vi "QCA Change Channels.vi"(0 "Channel":i32) -> ()   [LabVIEW 2010]
uses:
  QCA Global.vi
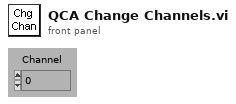
[diagram p1: front panel]
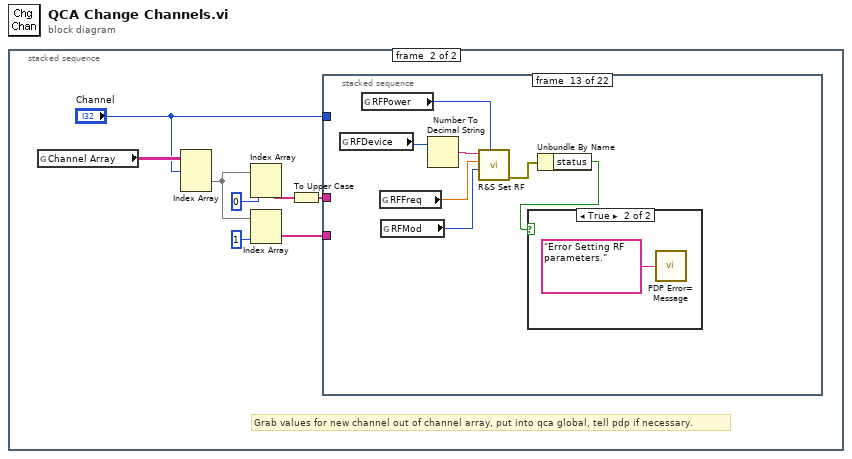
[diagram p0: block diagram]
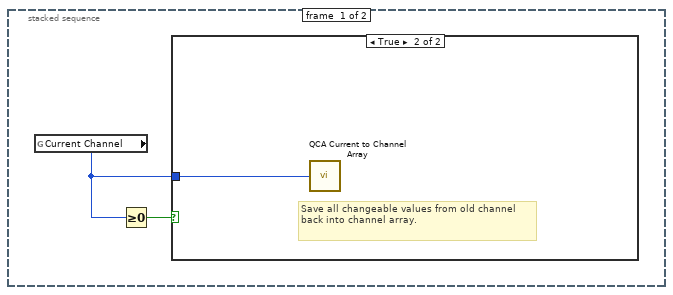
[diagram p2: hidden frame]
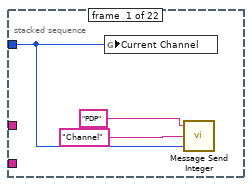
[diagram p4: hidden frame]
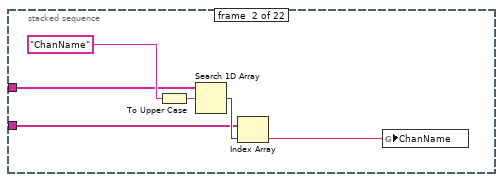
[diagram p5: hidden frame]
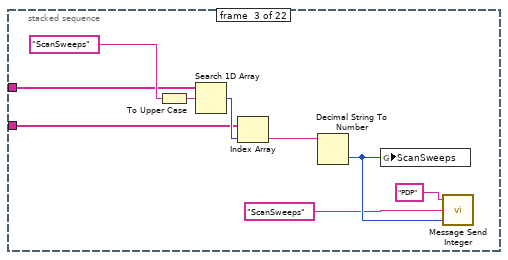
[diagram p6: hidden frame]
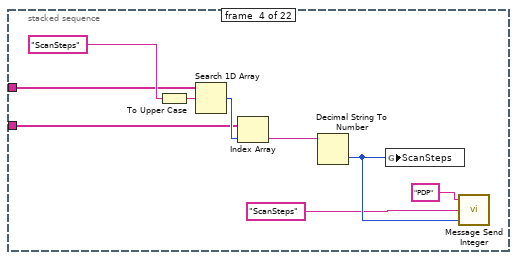
[diagram p7: hidden frame]
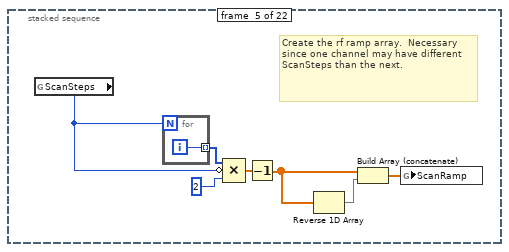
[diagram p8: hidden frame]
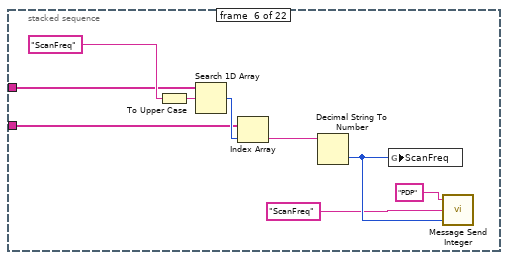
[diagram p9: hidden frame]
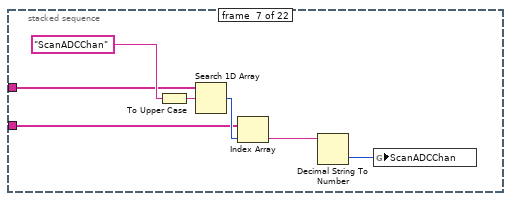
[diagram p10: hidden frame]
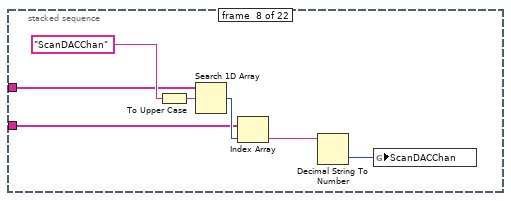
[diagram p11: hidden frame]
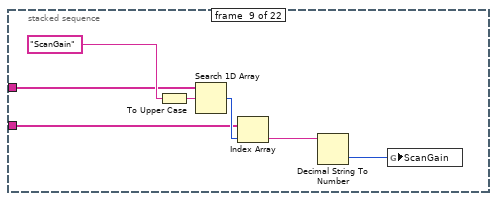
[diagram p12: hidden frame]
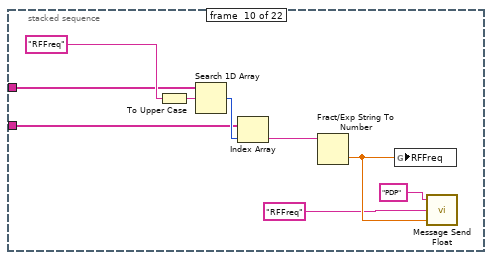
[diagram p13: hidden frame]
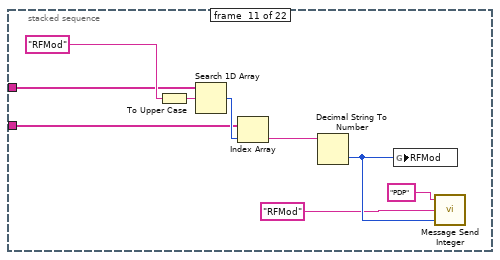
[diagram p14: hidden frame]
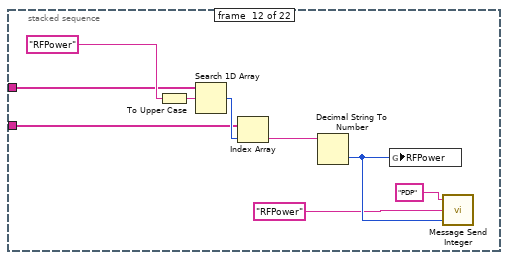
[diagram p15: hidden frame]
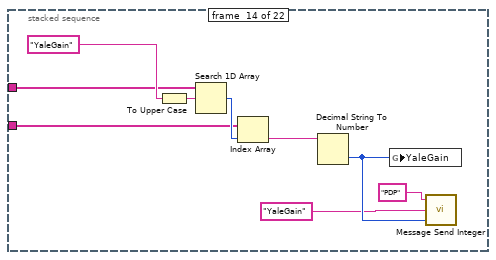
[diagram p17: hidden frame]
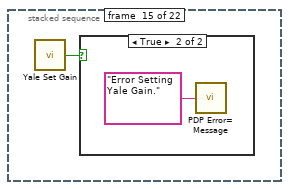
[diagram p18: hidden frame]
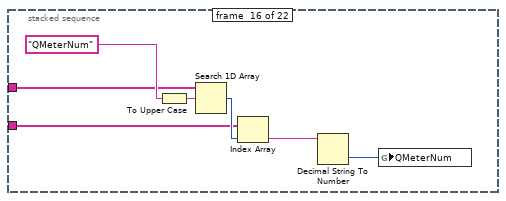
[diagram p20: hidden frame]
diagram:
  n1 = stacked-sequence {
    frame #0 {
      n2 = global read "QCA Global.vi" "Current Channel"() -> (w1:i32)
      n3 = Greater Or Equal To 0?(x=w1) -> (x >= 0?=w2:bool)
      n4 = case shown="True" w2 {
        tunnel: w1 -> [_ w3]
        frame False {
        }
        frame True {
          # "Save all changeable values from old channel back into channel array."
          n5 = call "QCA Current to Channel Array.vi"("Channel Number"=w3) -> ()
        }
      }
    }
    frame #1 {
      # "Grab values for new channel out of channel array, put into qca global, tell pdp if necessary."
      n6 = global read "QCA Global.vi" "Channel Array"() -> (w10:string[][][])
      n7 = Index Array(array=w10, index (dim 0)="Channel") -> (element=w6:string[][])  [unwired: 2 in]
      n8 = Index Array(array=w6, index (col)=0 ("Index")) -> (element=w9:string[])  [unwired: 1 in]
      n9 = Index Array(array=w6, index (col)=1 ("Index")) -> (element=w7:string[])  [unwired: 1 in]
      n10 = To Upper Case(1:w9) -> (0:w4:string[])
      n11 = stacked-sequence {
        tunnel: w4 -> [_ w17 w26 w35 _ w52 w59 w66 w73 w82 w91 w100 _ w117 _ w126 w134 _ w145 w155 w166 w173]
        tunnel: w7 -> [_ w16 w25 w34 _ w51 w58 w65 w72 w81 w90 w99 _ w116 _ w125 w133 _ w144 w154 w165 w172]
        tunnel: "Channel" -> [w14 _ _ _ _ _ _ _ _ _ _ _ _ _ _ _ _ _ _ _ _ _]
        frame #0 {
          n12 = global write "QCA Global.vi" "Current Channel"(w14) -> ()
          n13 = call "Message Send Integer.vi"("Value"=w14, "Parameter"="Channel", "Destination"="PDP") -> ()
        }
        frame #1 {
          n14 = To Upper Case(1:"ChanName" ("element")) -> (0:w18:string)
          n15 = Search 1D Array(1D array=w17, element=w18) -> (index of element=w19:i32)  [unwired: 1 in]
          n16 = Index Array(array=w16, index=w19) -> (element=w15:string)
          n17 = global write "QCA Global.vi" "ChanName"(w15) -> ()
        }
        frame #2 {
          n18 = To Upper Case(1:"ScanSweeps" ("element")) -> (0:w27:string)
          n19 = Search 1D Array(1D array=w26, element=w27) -> (index of element=w28:i32)  [unwired: 1 in]
          n20 = Index Array(array=w25, index=w28) -> (element=w24:string)
          n21 = Decimal String To Number(string=w24) -> (number=w23:i32)  [unwired: 2 in, 1 out]
          n22 = global write "QCA Global.vi" "ScanSweeps"(w23) -> ()
          n23 = call "Message Send Integer.vi"("Value"=w23, "Parameter"="ScanSweeps", "Destination"="PDP") -> ()
        }
        frame #3 {
          n24 = To Upper Case(1:"ScanSteps" ("element")) -> (0:w36:string)
          n25 = Search 1D Array(1D array=w35, element=w36) -> (index of element=w37:i32)  [unwired: 1 in]
          n26 = Index Array(array=w34, index=w37) -> (element=w33:string)
          n27 = Decimal String To Number(string=w33) -> (number=w32:i32)  [unwired: 2 in, 1 out]
          n28 = global write "QCA Global.vi" "ScanSteps"(w32) -> ()
          n29 = call "Message Send Integer.vi"("Value"=w32, "Parameter"="ScanSteps", "Destination"="PDP") -> ()
        }
        frame #4 {
          # "Create the rf ramp array.  Necessary since one channel may have different ScanSteps than the next."
          n30 = global read "QCA Global.vi" "ScanSteps"() -> (w42:i32)
          n31 = for {
            N: w42 -> [_]
            tunnel: [w46] -> w45 mode=indexing
            i -> [w46]
          }
          n32 = Compound Arithmetic op=MULTIPLY(w45, invert w42, 2 ("Input")) -> (w43:dbl[])
          n33 = Decrement(x=w43) -> (x-1=w40:dbl[])
          n34 = Reverse 1D Array(array=w40) -> (reversed array=w41:dbl[])
          n35 = Build Array (concatenate)(w40, w41) -> (w39:dbl[])
          n36 = global write "QCA Global.vi" "ScanRamp"(w39) -> ()
        }
        frame #5 {
          n37 = To Upper Case(1:"ScanFreq" ("element")) -> (0:w53:string)
          n38 = Search 1D Array(1D array=w52, element=w53) -> (index of element=w54:i32)  [unwired: 1 in]
          n39 = Index Array(array=w51, index=w54) -> (element=w50:string)
          n40 = Decimal String To Number(string=w50) -> (number=w49:i32)  [unwired: 2 in, 1 out]
          n41 = global write "QCA Global.vi" "ScanFreq"(w49) -> ()
          n42 = call "Message Send Integer.vi"("Value"=w49, "Parameter"="ScanFreq", "Destination"="PDP") -> ()
        }
        frame #6 {
          n43 = To Upper Case(1:"ScanADCChan" ("element")) -> (0:w60:string)
          n44 = Search 1D Array(1D array=w59, element=w60) -> (index of element=w61:i32)  [unwired: 1 in]
          n45 = Index Array(array=w58, index=w61) -> (element=w57:string)
          n46 = Decimal String To Number(string=w57) -> (number=w56:i32)  [unwired: 2 in, 1 out]
          n47 = global write "QCA Global.vi" "ScanADCChan"(w56) -> ()
        }
        frame #7 {
          n48 = To Upper Case(1:"ScanDACChan" ("element")) -> (0:w67:string)
          n49 = Search 1D Array(1D array=w66, element=w67) -> (index of element=w68:i32)  [unwired: 1 in]
          n50 = Index Array(array=w65, index=w68) -> (element=w64:string)
          n51 = Decimal String To Number(string=w64) -> (number=w63:i32)  [unwired: 2 in, 1 out]
          n52 = global write "QCA Global.vi" "ScanDACChan"(w63) -> ()
        }
        frame #8 {
          n53 = To Upper Case(1:"ScanGain" ("element")) -> (0:w74:string)
          n54 = Search 1D Array(1D array=w73, element=w74) -> (index of element=w75:i32)  [unwired: 1 in]
          n55 = Index Array(array=w72, index=w75) -> (element=w71:string)
          n56 = Decimal String To Number(string=w71) -> (number=w70:i32)  [unwired: 2 in, 1 out]
          n57 = global write "QCA Global.vi" "ScanGain"(w70) -> ()
        }
        frame #9 {
          n58 = To Upper Case(1:"RFFreq" ("element")) -> (0:w83:string)
          n59 = Search 1D Array(1D array=w82, element=w83) -> (index of element=w84:i32)  [unwired: 1 in]
          n60 = Index Array(array=w81, index=w84) -> (element=w80:string)
          n61 = Fract/Exp String To Number(string=w80) -> (number=w79:dbl)  [unwired: 3 in, 1 out]
          n62 = global write "QCA Global.vi" "RFFreq"(w79) -> ()
          n63 = call "Message Send Float.vi"("Value"=w79, "Parameter"="RFFreq", "Destination"="PDP") -> ()
        }
        frame #10 {
          n64 = To Upper Case(1:"RFMod" ("element")) -> (0:w92:string)
          n65 = Search 1D Array(1D array=w91, element=w92) -> (index of element=w93:i32)  [unwired: 1 in]
          n66 = Index Array(array=w90, index=w93) -> (element=w89:string)
          n67 = Decimal String To Number(string=w89) -> (number=w88:i32)  [unwired: 2 in, 1 out]
          n68 = global write "QCA Global.vi" "RFMod"(w88) -> ()
          n69 = call "Message Send Integer.vi"("Value"=w88, "Parameter"="RFMod", "Destination"="PDP") -> ()
        }
        frame #11 {
          n70 = To Upper Case(1:"RFPower" ("element")) -> (0:w101:string)
          n71 = Search 1D Array(1D array=w100, element=w101) -> (index of element=w102:i32)  [unwired: 1 in]
          n72 = Index Array(array=w99, index=w102) -> (element=w98:string)
          n73 = Decimal String To Number(string=w98) -> (number=w97:i32)  [unwired: 2 in, 1 out]
          n74 = global write "QCA Global.vi" "RFPower"(w97) -> ()
          n75 = call "Message Send Integer.vi"("Value"=w97, "Parameter"="RFPower", "Destination"="PDP") -> ()
        }
        frame #12 {
          n76 = global read "QCA Global.vi" "RFDevice"() -> (w106:i32)
          n77 = global read "QCA Global.vi" "RFPower"() -> (w108:i32)
          n78 = global read "QCA Global.vi" "RFFreq"() -> (w109:dbl)
          n79 = global read "QCA Global.vi" "RFMod"() -> (w110:i32)
          n80 = Number To Decimal String(number=w106) -> (decimal integer string=w107:string)  [unwired: 1 in]
          n81 = call "R&S Set RF.vi"("amplitude (mV)"=w108, "modulation (kHz)"=w110, "center frequency (MHz)"=w109, "address"=w107) -> ("error out"=w105:errorcluster)  [unwired: 3 in, 1 out]
          n82 = Unbundle By Name(w105) -> ("status"=w104:bool)
          n83 = case shown="True" w104 {
            frame False {
            }
            frame True {
              n84 = call "PDP Error= Message.vi"("Message"="Error Setting RF parameters.") -> ()
            }
          }
        }
        frame #13 {
          n85 = To Upper Case(1:"YaleGain" ("element")) -> (0:w118:string)
          n86 = Search 1D Array(1D array=w117, element=w118) -> (index of element=w119:i32)  [unwired: 1 in]
          n87 = Index Array(array=w116, index=w119) -> (element=w115:string)
          n88 = Decimal String To Number(string=w115) -> (number=w114:i32)  [unwired: 2 in, 1 out]
          n89 = global write "QCA Global.vi" "YaleGain"(w114) -> ()
          n90 = call "Message Send Integer.vi"("Value"=w114, "Parameter"="YaleGain", "Destination"="PDP") -> ()
        }
        frame #14 {
          n91 = call "Yale Set Gain.vi"() -> ("Error"=w121:bool)
          n92 = case shown="True" w121 {
            frame False {
            }
            frame True {
              n93 = call "PDP Error= Message.vi"("Message"="Error Setting Yale Gain.") -> ()
            }
          }
        }
        frame #15 {
          n94 = To Upper Case(1:"QMeterNum" ("element")) -> (0:w127:string)
          n95 = Search 1D Array(1D array=w126, element=w127) -> (index of element=w128:i32)  [unwired: 1 in]
          n96 = Index Array(array=w125, index=w128) -> (element=w124:string)
          n97 = Decimal String To Number(string=w124) -> (number=w123:i32)  [unwired: 2 in, 1 out]
          n98 = global write "QCA Global.vi" "QMeterNum"(w123) -> ()
        }
        frame #16 {
          n99 = To Upper Case(1:"QMeterName" ("element")) -> (0:w135:string)
          n100 = Search 1D Array(1D array=w134, element=w135) -> (index of element=w136:i32)  [unwired: 1 in]
          n101 = Index Array(array=w133, index=w136) -> (element=w132:string)
          n102 = global write "QCA Global.vi" "QMeterName"(w132) -> ()
          n103 = call "Message Send Text.vi"("Value"=w132, "Parameter"="QMeterName", "Destination"="PDP") -> ()
        }
        frame #17 {
          n104 = call "QMeter Select.vi"() -> ("Error"=w138:bool)
          n105 = case shown="True" w138 {
            frame False {
            }
            frame True {
              n106 = call "PDP Error= Message.vi"("Message"="Error Selecting QMeter.") -> ()
            }
          }
        }
        frame #18 {
          n107 = To Upper Case(1:"CalConst" ("element")) -> (0:w146:string)
          n108 = Search 1D Array(1D array=w145, element=w146) -> (index of element=w147:i32)  [unwired: 1 in]
          n109 = Index Array(array=w144, index=w147) -> (element=w143:string)
          n110 = Fract/Exp String To Number(string=w143) -> (number=w142:dbl)  [unwired: 3 in, 1 out]
          n111 = global write "QCA Global.vi" "CalConst"(w142) -> ()
          n112 = call "Message Send Float.vi"("Value"=w142, "Parameter"="CalConst", "Destination"="PDP") -> ()
        }
        frame #19 {
          n113 = To Upper Case(1:"Baseline" ("element")) -> (0:w156:string)
          n114 = Search 1D Array(1D array=w155, element=w156) -> (index of element=w157:i32)  [unwired: 1 in]
          n115 = Index Array(array=w154, index=w157) -> (element=w153:string)
          n116 = Decimal String To Number(string=w153) -> (number=w149:i32)  [unwired: 2 in, 1 out]
          n117 = case shown="1, Default" w149 {
            tunnel: w149 -> [_ _ w162]
            tunnel: ["New Baseline" ("TimeStamp") "No Baseline" ("TimeStamp") w161] -> w152
            frame 0 {
            }
            frame -1 {
            }
            frame 1, Default {
              n118 = call "Event Number to Timestamp.vi"("Event Number"=w162) -> ("TimeStamp"=w161:string)
            }
          }
          n119 = global write "QCA Global.vi" "Baseline"(w149) -> ()
          n120 = call "Message Send Text.vi"("Value"=w152, "Parameter"="Baseline", "Destination"="PDP") -> ()
        }
        frame #20 {
          n121 = To Upper Case(1:"DCLevelChan" ("element")) -> (0:w167:string)
          n122 = Search 1D Array(1D array=w166, element=w167) -> (index of element=w168:i32)  [unwired: 1 in]
          n123 = Index Array(array=w165, index=w168) -> (element=w164:string)
          n124 = Decimal String To Number(string=w164) -> (number=w163:i32)  [unwired: 2 in, 1 out]
          n125 = global write "QCA Global.vi" "DCLevelChan"(w163) -> ()
        }
        frame #21 {
          n126 = To Upper Case(1:"QMeterTempChan" ("element")) -> (0:w174:string)
          n127 = Search 1D Array(1D array=w173, element=w174) -> (index of element=w175:i32)  [unwired: 1 in]
          n128 = Index Array(array=w172, index=w175) -> (element=w171:string)
          n129 = Decimal String To Number(string=w171) -> (number=w170:i32)  [unwired: 2 in, 1 out]
          n130 = global write "QCA Global.vi" "QMeterTempChan"(w170) -> ()
        }
      }
    }
  }
